vi "Klinger ControlLimit.vi"(0 "Axe":u8(ring) items=["W", "X", "Y", "Z"], 1 "UnitDem":u8(ring) caption="Unités\nDemandées" items=["Pas", "mm", "ps", "Degré (°)"], 3 "error in":errorcluster) -> (5 "DataRange":T1 {"Increment" format="%#_1g"; "Maximum" format="%#_10g"; "Minimum" format="%#_10g"}, 6 "FormtPrec":cluster{"Format":u8, "Precision":u8} caption="Format &\nPrécision", 7 "error out":errorcluster)   [LabVIEW 2010]
doc: "Ce VI retourne la plage des données acceptable par le contrôleur en fonction de l'axe et de l'unité choisi. Il retourne le maximum, le minimum, l'incrément (résolution), et la précision d'affichage à appliquer au contrôle de consigne de déplacement, pour l'axe et l'unité en vigueur. Cela empêche la saisi de consigne hors limite."
uses:
  <userlib>/Klinger/Klinger Lib.llb/Klinger ConvUnitArr.vi
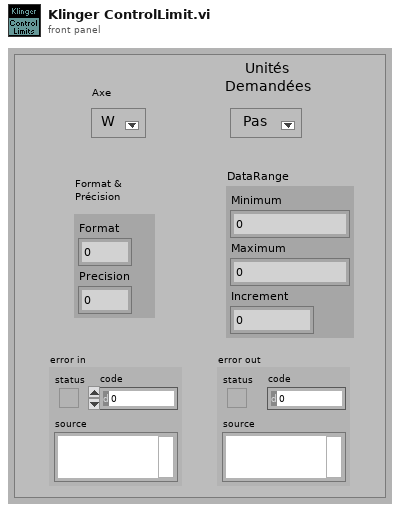
[diagram p1: front panel]
types:
  T1 = cluster{"Minimum":dbl, "Maximum":dbl, "Increment":dbl}
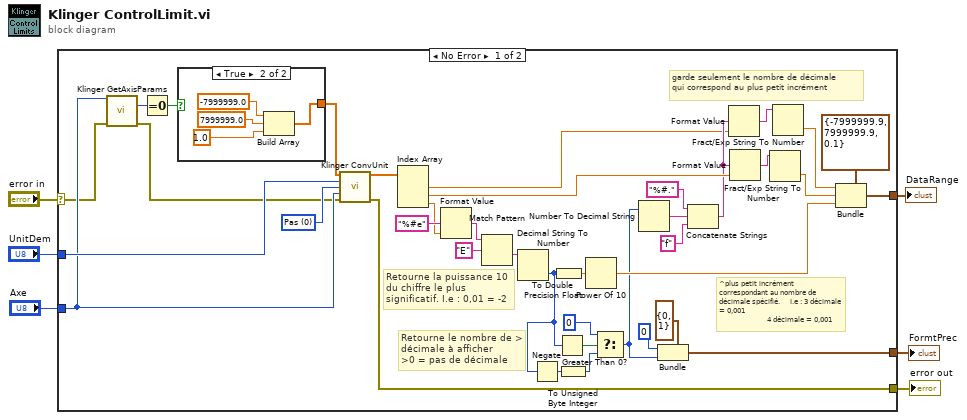
[diagram p0: block diagram]
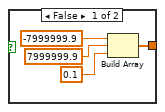
[diagram p2: hidden frame]
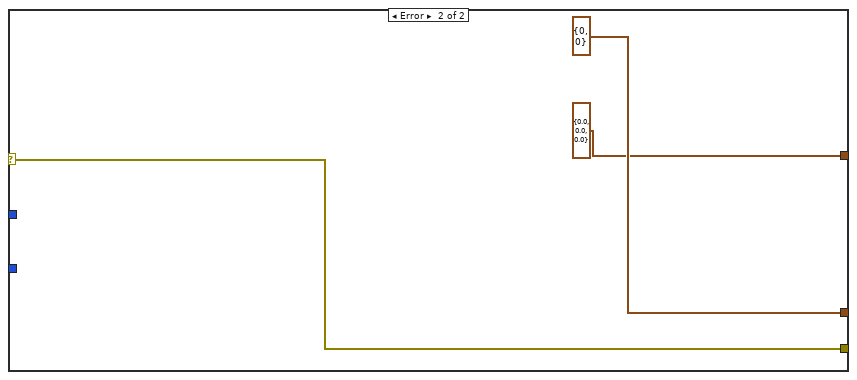
[diagram p3: hidden frame]
diagram:
  n1 = case shown="No Error" "error in" {
    selector: "error in" -> [w36 w55]
    tunnel: [w43 w55] -> w6
    tunnel: "Axe" -> [w40 _]
    tunnel: "UnitDem" -> [w42 _]
    tunnel: [w34 T1 {"Minimum"=0.0, "Maximum"=0.0, "Increment"=0.0} ("Data Range")] -> w2
    tunnel: [w31 cluster{"Format":u8, "Precision":u8} {"Format"=0, "Precision"=0} ("Format & Precision")] -> w1
    frame No Error {
      w41 = u8 0 items=["Pas", "mm", "ps", "Degré (°)"] ("UnitAct")
      # "Retourne la puissance 10\ndu chiffre le plus significatif. I.e : 0,01 = -2"
      # "^plus petit incrément correspondant au nombre de décimale spécifié.     I.e : 3 décimale = 0,001\n                        4 décimale = 0,001"
      # "Retourne le nombre de > décimale à afficher\n>0 = pas de décimale"
      # "garde seulement le nombre de décimale\nqui correspond au plus petit incrément"
      n2 = call <userlib>:"Klinger GetAxisParams.vi"("Axe"=w40, "error in"=w36) -> ("Type"=w39:i32, "error out"=w35:errorcluster)  [unwired: 6 in, 6 out]
      n3 = Equal To 0?(x=w39) -> (x = 0?=w38:bool)
      n4 = case shown="True" w38 {
        tunnel: [w45 w49] -> w37
        frame False {
          n5 = Build Array(-7999999.9 ("Minimum"), 7999999.9 ("Maximum"), 0.1 ("Increment")) -> (w45:dbl[])
        }
        frame True {
          n6 = Build Array(-7999999.0 ("Minimum"), 7999999.0 ("Minimum"), 1.0 ("Increment")) -> (w49:dbl[])
        }
      }
      n7 = call-poly <userlib>:"Klinger ConvUnit.vi"("ParamAct"=w37, "UnitDem"=w42, "UnitAct"=w41, "Axe"=w40, "error in"=w35) -> ("ParamDem"=w30:dbl[], "error out"=w43:errorcluster)  [unwired: 9 in]
      n8 = Index Array(array=w30) -> (element #1=w18:dbl, element #2=w25:dbl, element #3=w26:dbl)  [unwired: 3 in]
      n9 = Format Value(format string="%#e", value (0)=w26) -> (output string=w27:string)  [unwired: 1 in]
      n10 = Match Pattern(string=w27, regular expression="E") -> (after substring=w14:string)  [unwired: 1 in, 3 out]
      n11 = Decimal String To Number(string=w14) -> (number=w8:i32)  [unwired: 2 in, 1 out]
      n12 = Negate(x=w8) -> (-x=w10:i32)
      n13 = To Double Precision Float(number=w8) -> (double precision float=w21:dbl)
      n14 = Greater Than 0?(x=w8) -> (x > 0?=w12:bool)
      n15 = To Unsigned Byte Integer(number=w10) -> (unsigned 8bit integer=w9:u8)
      n16 = Power Of 10(x=w21) -> (10^x=w13:dbl)
      n17 = Select(t=u8 0 ("Format"), s=w12, f=w9) -> (s? t:f=w7:u8)
      n18 = Number To Decimal String(number=w7) -> (decimal integer string=w20:string)  [unwired: 1 in]
      n19 = Bundle(cluster=cluster{"Format":u8, "Precision":u8} {"Format"=0, "Precision"=1} ("Format & Precision"), "Format"=u8 0, "Precision"=w7) -> (w31:cluster{"Format":u8, "Precision":u8})
      n20 = Concatenate Strings("%#." ("format string"), w20, "f" ("format string")) -> (w19:string)
      n21 = Format Value(format string=w19, value (0)=w18) -> (output string=w17:string)  [unwired: 1 in]
      n22 = Format Value(format string=w19, value (0)=w25) -> (output string=w16:string)  [unwired: 1 in]
      n23 = Fract/Exp String To Number(string=w16) -> (number=w24:dbl)  [unwired: 3 in, 1 out]
      n24 = Fract/Exp String To Number(string=w17) -> (number=w15:dbl)  [unwired: 3 in, 1 out]
      n25 = Bundle(cluster=T1 {"Minimum"=-7999999.9, "Maximum"=7999999.9, "Increment"=0.1} ("Data Range"), "Minimum"=w15, "Maximum"=w24, "Increment"=w13) -> (w34:T1)
    }
    frame Error {
    }
  }
  "error out" <- w6
  "DataRange" <- w2
  "FormtPrec" <- w1
